vi "Read Events.vi"(11 "Status Updater in":refnum<class "Status Updater.lvclass">) -> (2 "Status Events":refnum<class "Status Events.lvclass">)   [LabVIEW 2014, in "Status Updater.lvclass"]
uses:
  Status Updater.lvclass
  Status Events/Status Events.lvclass
  Status Updater.lvclass/Status Updater.ctl
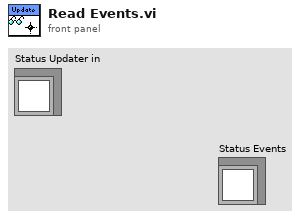
[diagram p1: front panel]
types:
  T1 = cluster{"Build Text":refnum<user-event>, "Progress":refnum<user-event>}
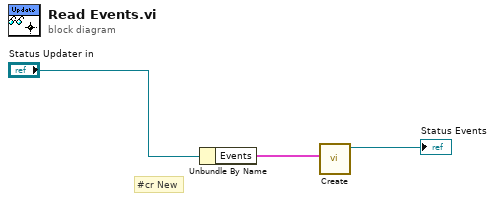
[diagram p0: block diagram]
diagram:
  # "#cr New"
  n1 = Unbundle By Name("Status Updater in") -> ("Events"=w2:T1)
  n2 = call "Create.vi"("Events"=w2) -> ("Status Updater out"=→"Status Events":refnum<class "Status Events.lvclass">)  [unwired: 10 in]
